vi "RT_9073_Load_Cell.vi"() -> ()   [LabVIEW 2019]
uses:
  <vilib>/userDefined/High Color/nirio_resource_hc.ctl
  Type Def/nicrio_cRIO-9237_DataRatesRing.ctl
  Type Def/nicrio_cRIO-9237_ExcitationVoltageRing.ctl
  <vilib>/FPGAPlugInAG/cRIO-9073/niLvFpga_Open_cRIO-9073.vi
  <vilib>/rvi/interface/common/dynamic/niFpgaDynamicAddResources.vi
  <vilib>/Utility/error.llb/Error Cluster From Error Code.vi
  <vilib>/rvi/errors/niLvFpgaAdjustHostInterfaceError.vi
  <vilib>/FPGAPlugInAG/Dynamic/niLvFpga_Close_Dynamic.vi
  <vilib>/rvi/interface/nirviOpenFPGA/nirviOpenFPGA.xnode
  On Call Bitfiles/gpass2home_FPGATarget_crio9073FPGALoad_XTL2lUff-PU.lvbitx
  <vilib>/rvi/interface/nirviReadWriteControl/nirviReadWriteControl.xnode
  <vilib>/rvi/interface/nirviCloseFPGA/nirviCloseFPGA.xnode
  NiFpgaLv.dll
  <vilib>/rvi/interface/Simulation/niFpgaSimulationCallBeginRW.vi
panel:
  in  "Excitation Voltage":T1 items=["2.5 Volts", "3.3 Volts", "5.0 Volts", "10.0 Volts", "External Excitation"]
  in  "Data Rate":T2=1 items=["50.000 kS/s (NI 9237)"=1, "25.000 kS/s (NI 9237)"=2, "16.667 kS/s (NI 9237)"=3, "12.500 kS/s (NI 9237)"=4, "10.000 kS/s (NI 9237)"=5, "8.333 kS/s (NI 9237)"=6, "7.143 kS/s (NI 9237)"=7, "6.250 kS/s (NI 9237)"=8, "5.556 kS/s (NI 9237)"=9, "5.000 kS/s (NI 9237)"=10, "4.545 kS/s (NI 9237)"=11, "4.167 kS/s (NI 9237)"=12, "3.846 kS/s (NI 9237)"=13, "3.571 kS/s (NI 9237)"=14, "3.333 kS/s (NI 9237)"=15, "3.125 kS/s (NI 9237)"=16, "2.941 kS/s (NI 9237)"=17, "2.778 kS/s (NI 9237)"=18, "2.632 kS/s (NI 9237)"=19, "2.500 kS/s (NI 9237)"=20, "2.381 kS/s (NI 9237)"=21, "2.273 kS/s (NI 9237)"=22, "2.174 kS/s (NI 9237)"=23, "2.083 kS/s (NI 9237)"=24, "2.000 kS/s (NI 9237)"=25, "1.923 kS/s (NI 9237)"=26, "1.852 kS/s (NI 9237)"=27, "1.786 kS/s (NI 9237)"=28, "1.724 kS/s (NI 9237)"=29, "1.667 kS/s (NI 9237)"=30, "1.613 kS/s (NI 9237)"=31]
  in  "resource name":T3="RIO0"
  in  "stop":bool
  out "Mod1/AI0":fxp<+/-,24,-4>
  in  "Finite ?":bool
  in  "Shunt Cal Enable":bool
  in  "Half-Bridge Enable":bool
  in  "Loop Rate (uSec)":u32=100
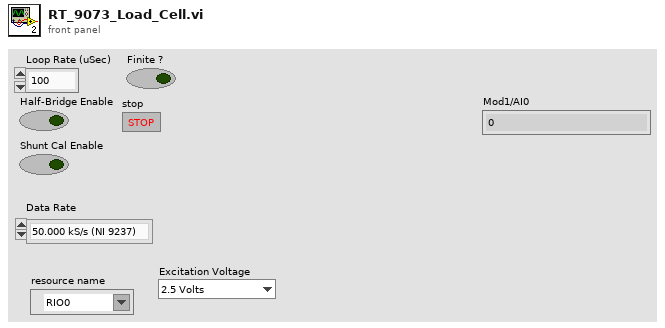
[diagram p1: front panel]
types:
  T1 = typedef "nicrio_cRIO-9237_ExcitationVoltageRing.ctl" = u8
  T2 = typedef "nicrio_cRIO-9237_DataRatesRing.ctl" = u8
  T3 = typedef "nirio_resource_hc.ctl" = tag
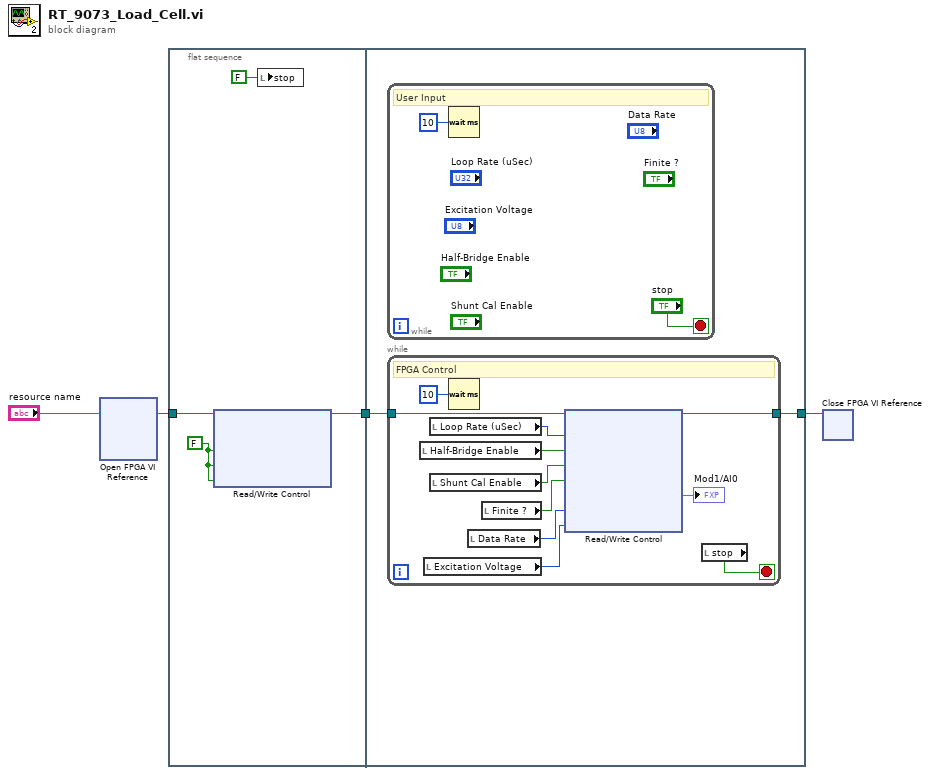
[diagram p0: block diagram]
diagram:
  n1 = xnode "Open FPGA VI Reference"("resource name"="resource name") -> ("FPGA VI Reference Out"=w4:refnum<k20>)  [unwired: 1 in, 1 out]
  n2 = flat-sequence {
    tunnel: w4 -> [w8]
    tunnel: [w5] -> w3
    tunnel: w3 -> [w10]
    tunnel: [w9] -> w2
    frame #0 {
      w7 = FALSE ("Half-Bridge Enable")
      n3 = xnode "Read/Write Control"("FPGA VI Reference In"=w8, "Half-Bridge Enable"=w7, "Shunt Cal Enable"=w7, "Finite?"=w7) -> ("FPGA VI Reference Out"=w5:refnum<k20>)  [unwired: 2 in, 1 out]
      n4 = local write "stop"(FALSE ("stop")) -> ()
    }
    frame #1 {
      n5 = while {
        stop <- "stop" stop-if-true
        # "User Input"
        n6 = Wait (ms)(milliseconds to wait=u32 10) -> ()  [unwired: 1 out]
      }
      n7 = while {
        tunnel: w10 -> [w17]
        tunnel: [w16] -> w9
        stop <- w18 stop-if-true
        # "FPGA Control"
        n8 = local read "Half-Bridge Enable"() -> (w22:bool)
        n9 = local read "Excitation Voltage"() -> (w14:T1)
        n10 = local read "Loop Rate (uSec)"() -> (w23:u32)
        n11 = local read "Shunt Cal Enable"() -> (w21:bool)
        n12 = Wait (ms)(milliseconds to wait=u32 10) -> ()  [unwired: 1 out]
        n13 = local read "Data Rate"() -> (w15:T2)
        n14 = local read "Finite ?"() -> (w20:bool)
        n15 = xnode "Read/Write Control"("FPGA VI Reference In"=w17, "Loop Rate (uSec)"=w23, "Half-Bridge Enable"=w22, "Shunt Cal Enable"=w21, "Finite?"=w20, "Data Rate"=w15, "Excitation Voltage"=w14) -> ("FPGA VI Reference Out"=w16:refnum<k20>, "Mod1/AI0"=→"Mod1/AI0":fxp<+/-,24,-4>)  [unwired: 1 in, 1 out]
        n16 = local read "stop"() -> (w18:bool)
      }
    }
  }
  n17 = xnode "Close FPGA VI Reference"("FPGA VI Reference In"=w2) -> ()  [unwired: 1 in, 1 out]
